vi "test_MultipleSessionsReserved_CallCloseSessionsWithErrorInput_ConnectionMapSessionsCleared.vi"(8 "error in":errorcluster) -> (0 "error out":errorcluster, 2 "result":string, 3 "pass":bool)   [LabVIEW 2020, in "MeasurementServerTests.lvlib"]
uses:
  MeasurementServerTests.lvlib
  Runtime/MeasurementLink Session Management/Session Reservation/Session Reservation.lvclass
  1bc5ef01-1aeb-4a5a-947f-0a0029d5b893.vi
  Runtime/MeasurementLink Session Management/Session Reservation/Connection.ctl
  Runtime/MeasurementLink Session Management/Session Reservation/Connection with Session.ctl
  473e7f0a-8276-4b7e-9ee7-44a9c5d89e8b.vi
  Helpers/Fake Instrument/Fake Instrument.lvclass
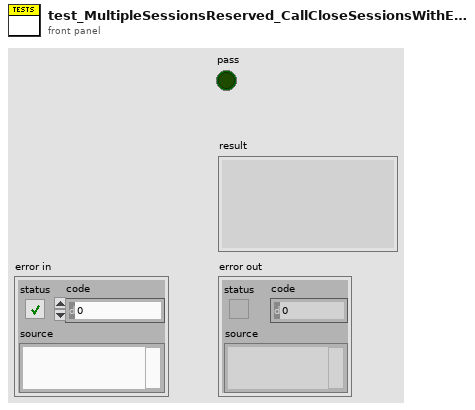
[diagram p1: front panel]
types:
  T1 = typedef "MeasurementLink Session Management.lvlib/Session Reservation.lvclass/Connection with Session.ctl" = cluster{"connection":T2, "session":variant}
  T2 = typedef "MeasurementLink Session Management.lvlib/Session Reservation.lvclass/Connection.ctl" = cluster{"pin or relay name":string, "site":i32, "instrument type id":string, "channel":string}
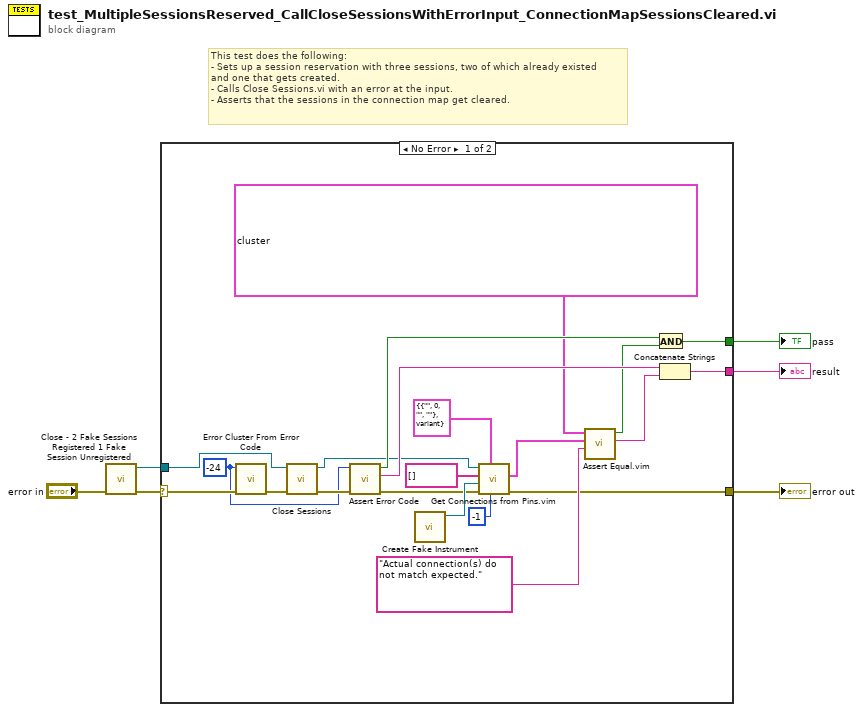
[diagram p0: block diagram]
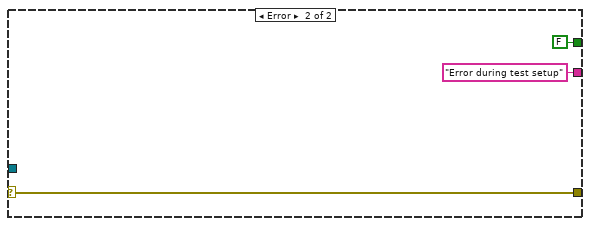
[diagram p2: hidden frame]
diagram:
  # "This test does the following:\n- Sets up a session reservation with three sessions, two of which already existed\nand one that gets created.\n- Calls Close Sessions.vi with an error at the input.\n- Asserts that the sessions in the connection map get cleared."
  n1 = call "Close - 2 Fake Sessions Registered 1 Fake Session Unregistered.vi"("error in (no error)"="error in") -> ("error out"=w5:errorcluster, "Session Reservation out"=w4:refnum<class "Session Reservation.lvclass">)  [unwired: 9 in]
  n2 = case shown="No Error" w5 {
    selector: w5 -> [w25 w29]
    tunnel: w4 -> [w27 _]
    tunnel: [w9 w29] -> w3
    tunnel: [w22 FALSE ("pass")] -> w2
    tunnel: [w20 "Error during test setup" ("result")] -> w1
    frame No Error {
      w23 = -24 ("error code (0)")
      n3 = call <vilib>:"Error Cluster From Error Code.vi"("error in (no error)"=w25, "error code (0)"=w23) -> ("error out"=w24:errorcluster)  [unwired: 7 in]
      n4 = call "Close Sessions.vi"("error in"=w24, "session reservation in"=w27) -> ("error out"=w26:errorcluster, "session reservation out"=w10:refnum<class "Session Reservation.lvclass">)  [unwired: 8 in]
      n5 = call "Assert Error Code.vi"("error in"=w26, "expected error code"=w23) -> ("error out"=w12:errorcluster, "details"=w19:string, "error code match?"=w21:bool)  [unwired: 7 in]
      n6 = call "Create Fake Instrument.vi"() -> ("fake instrument out"=w14:refnum<class "Fake Instrument.lvclass">)  [unwired: 10 in, 1 out]
      n7 = call "Get Connections from Pins.vim"("site"=-1, "connection type"=T1 {"connection"={"pin or relay name"="", "site"=0, "instrument type id"="", "channel"=""}, "session"=variant}, "error in"=w12, "instrument"=w14, "pin or relay names"=string[] [], "session reservation in"=w10) -> ("error out"=w9:errorcluster, "connections"=w16:T1[])  [unwired: 3 in, 1 out]
      n8 = call "Assert Equal.vim"("failure message"="Actual connection(s) do not match expected.", "actual value"=w16, "expected value"=T1[] [{"connection"={"pin or relay name"="PinA", "site"=4, "instrument type id"="fake_instrument_type", "channel"="1"}, "session"=variant}, {"connection"={"pin or relay name"="PinB", "site"=4, "instrument type id"="fake_instrument_type", "channel"="0"}, "session"=variant}, {"connection"={"pin or relay name"="PinC", "site"=4, "instrument type id"="fake_instrument_type", "channel"="2"}, "session"=variant}] ("connections")) -> ("message"=w7:string, "equal?"=w8:bool)  [unwired: 7 in]
      n9 = And(x=w21, y=w8) -> (x .and. y?=w22:bool)
      n10 = Concatenate Strings(w19, w7) -> (w20:string)
    }
    frame Error {
    }
  }
  "error out" <- w3
  "pass" <- w2
  "result" <- w1
